vi "tb_2 input multiplexer (Host).vi"() -> ()   [LabVIEW 2010]
panel:
  out "Output Data Valid Array":bool[][](array[boolean])
  out "Interchanged Data":i16[][](array[numeric])
  in  "Input Data Valid Array":bool[](array[boolean])=[FALSE, FALSE]
  in  "Input Data":i16[](array[numeric])=[0, 0]
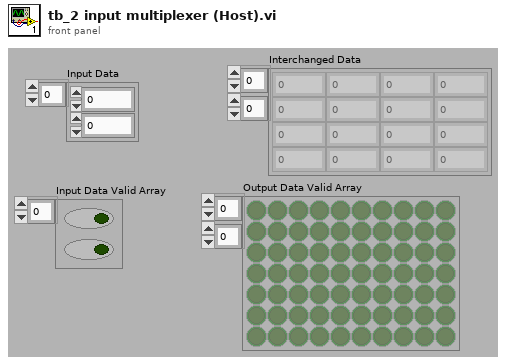
[diagram p1: front panel]
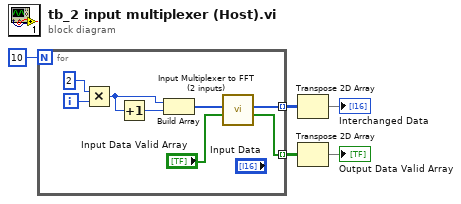
[diagram p0: block diagram]
diagram:
  n1 = for {
    N: 10 -> [_]
    tunnel: [w12] -> w5 mode=indexing
    tunnel: [w11] -> w3 mode=indexing
    i -> [w10]
    n2 = Multiply(x=2, y=w10) -> (x*y=w8:i32)
    n3 = Increment(x=w8) -> (x+1=w7:i32)
    n4 = Build Array(w8, w7) -> (w6:i32[])
    n5 = call "Input Multiplexer to FFT (2 inputs).vi"("Input Data Valid Array"="Input Data Valid Array", "Input Data"=w6) -> ("Output Data Valid Array"=w11:bool[], "Interchanged Data"=w12:i16[])  [unwired: 8 in]
  }
  n6 = Transpose 2D Array(2D array=w5) -> (transposed array=→"Interchanged Data":i16[][])
  n7 = Transpose 2D Array(2D array=w3) -> (transposed array=→"Output Data Valid Array":bool[][])
